vi "TestExec.Move File to New Folder.vi"(7 "Action":enum16{"Move", "Copy"}(ring), 8 "error in":errorcluster, 9 "ResultState":T1, 10 "Destination Folder":path, 11 "Source File Path":path) -> (0 "error out":errorcluster, 3 "New Path":path)   [LabVIEW 2018]
uses:
  <vilib>/KATE/SeqMgr/SeqMgr.Result State Enum.ctl
  Errors/Error.Error Code List.ctl
  <vilib>/KATE/Files/File Utils.lvlib
  <vilib>/KATE/SeqMgr/SeqMgr.lvlib
panel:
  out "Dir":bool
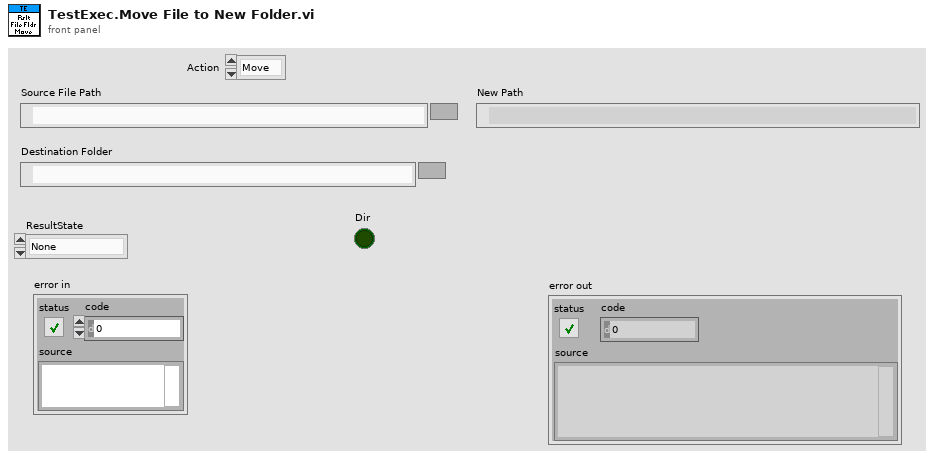
[diagram p1: front panel]
types:
  T1 = typedef "KATE_Lib.lvlib/SeqMgr.lvlib/SeqMgr.Result State Enum.ctl" = enum16{"None", "Passing", "Failing", "PASS", "FAIL", "ABORT", "ERROR"}
  T2 = typedef "Error.Error Code List.ctl" = i32
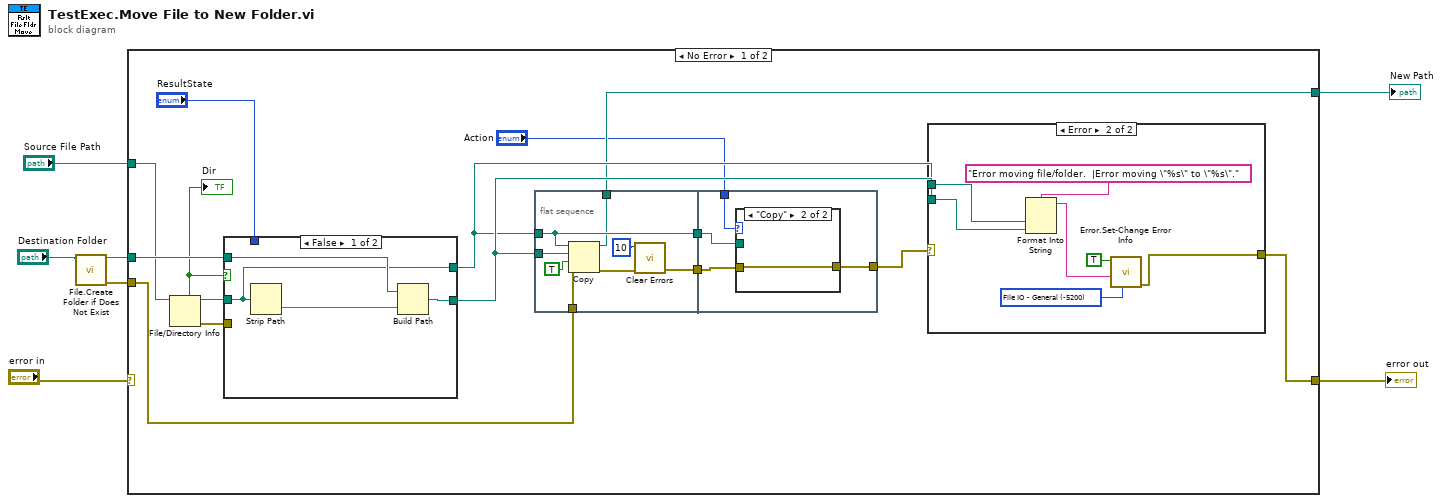
[diagram p0: block diagram]
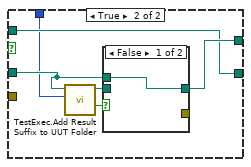
[diagram p2: hidden frame]
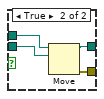
[diagram p3: hidden frame]
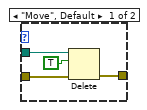
[diagram p4: hidden frame]
diagram:
  n1 = call <vilib>:"File.Create Folder if Does Not Exist.vi"("Path"="Destination Folder") -> ("error out"=w1:errorcluster, "Dup Path"=w3:path)  [unwired: 8 in, 1 out]
  n2 = case shown="No Error" "error in" {
    selector: "error in" -> [_ w62]
    tunnel: w3 -> [w22 _]
    tunnel: "Source File Path" -> [w12 _]
    tunnel: [w21 w62] -> w6
    tunnel: [w9 _] -> w5
    tunnel: w1 -> [w14 _]
    frame No Error {
      n3 = File/Directory Info(path=w12) -> (path out=w17:path, directory=w16:bool, error out=w15:errorcluster)  [unwired: 1 in, 4 out]
      "Dir" <- w16
      n4 = case shown="False" w16 {
        tunnel: w22 -> [w25 w29]
        tunnel: [w24 w29] -> w13
        tunnel: w17 -> [w23 w28]
        tunnel: w15 -> [_ _]
        tunnel: [w23 w30] -> w11
        tunnel: "ResultState" -> [_ w27]
        frame False {
          n5 = Strip Path(path=w23) -> (name=w26:string)  [unwired: 1 out]
          n6 = Build Path(base path=w25, name or relative path=w26) -> (appended path=w24:path)
        }
        frame True {
          n7 = call "TestExec.Add Result Suffix to UUT Folder.vi"("ResultState"=w27, "Path"=w28) -> ("Changed"=w32:bool, "New Path"=w31:path)  [unwired: 8 in]
          n8 = case shown="False" w32 {
            tunnel: w28 -> [w33 w37]
            tunnel: w31 -> [_ w36]
            tunnel: [w33 w35] -> w30
            tunnel: [_ w34] -> _
            frame False {
            }
            frame True {
              n9 = Move(source path=w37, 10:w36) -> (error out=w34:errorcluster, 3:w35:path)  [unwired: 3 in, 1 out]
            }
          }
        }
      }
      n10 = flat-sequence {
        tunnel: w11 -> [w44]
        tunnel: w13 -> [w45]
        tunnel: [w44] -> w20
        tunnel: [w43] -> w18
        tunnel: w14 -> [w39]
        tunnel: [w38] -> w9
        tunnel: w20 -> [w49]
        tunnel: [w47] -> w19
        tunnel: w18 -> [w48]
        tunnel: "Action" -> [w46]
        frame #0 {
          n11 = Copy(8:w39, 9:TRUE ("overwrite (F)"), 10:w45, 11:w44) -> (0:w42:errorcluster, 3:w38:path)  [unwired: 1 in, 1 out]
          n12 = call <vilib>:"Clear Errors.vi"("error in (no error)"=w42, "specific error code to clear (0: all)"=10) -> ("error out"=w43:errorcluster)  [unwired: 4 in, 1 out]
        }
        frame #1 {
          n13 = case shown="\"Copy\"" w46 {
            tunnel: w49 -> [w53 _]
            tunnel: w48 -> [w51 w54]
            tunnel: [w50 w54] -> w47
            frame "Move", Default {
              n14 = Delete(path (use dialog)=w53, entire hierarchy (F)=TRUE, error in=w51) -> (error out=w50:errorcluster)  [unwired: 2 in, 2 out]
            }
            frame "Copy" {
            }
          }
        }
      }
      n15 = case shown="Error" w19 {
        tunnel: w11 -> [_ w61]
        tunnel: w13 -> [_ w60]
        tunnel: [_ w55] -> w21
        frame No Error {
        }
        frame Error {
          w57 = T2 -5200 items=["No Error"=0, "Abort"=-2, "Misc"=-5000, "Fixture Error"=-5100, "File IO - General"=-5200, "FIle IO - Config Error"=-5201, "Instrument - General"=-5300, "Instrument - Serial Com"=-5301, "Instrument - Camera"=-5302, "Instrument - PS"=-5303, "Instrument - Oscilloscope"=-5304, "Instrument - Function Gen"=-5305, "Instrument - Load"=-5306, "Instrument - Meter"=-5307, "Instrument - Power Control"=-5308, "Instrument - Motion"=-5309, "Instrument - RF"=-5310, "System Exe"=-5400, "Image Processing"=-5500, "Communication"=-5600, "Script - Syntax Error"=-6000, "Script - Invalid Name or Param"=-6100, "Script - Timeout"=-6200, "Invalid Data"=-6300, "FW Update Error"=-6500] ("Std Code")
          n16 = Format Into String(format string="Error moving file/folder.  |Error moving \"%s\" to \"%s\".", w61, w60) -> (resulting string=w56:string)  [unwired: 2 in, 1 out]
          n17 = call "Error.Set-Change Error Info.vi"("Std Code"=w57, "Description"=w56, "Set Error"=TRUE) -> ("error out"=w55:errorcluster)  [unwired: 8 in]
        }
      }
    }
    frame Error {
    }
  }
  "New Path" <- w5
  "error out" <- w6
